vi "M1M3SupportSimulator.vi"   [LabVIEW 2016]
uses:
  Common_FPGA_HealthAndStatus/DataTypes/HealthAndStatusSettings.ctl
  Common_FPGA_Timestamp/DataTypes/TimestampSettings.ctl
  Common_FPGA_HealthAndStatus/DataTypes/HealthAndStatusFIFOCopySettings.ctl
  Common_FPGA_Modbus/DataTypes/ModbusPortSettings.ctl
  FPGAMockHPILC/DataTypes/MockHPILCSettings.ctl
  Common_FPGA_Modbus/DataTypes/ModbusCRCSettings.ctl
  FPGAMockFAILC/DataTypes/MockFAILC1Settings.ctl
  FPGAMockFAILC/DataTypes/MockFAILC2Settings.ctl
  FPGAMockFAILC/DataTypes/MockFAILC3Settings.ctl
  FPGAMockFAILC/DataTypes/MockFAILC4Settings.ctl
  FPGAMockInclin/DataTypes/MockInclinSettings.ctl
  FPGAMockDisplace/DataTypes/MockDisplaceSettings.ctl
  <vilib>/rvi/Emulation/niFpgaGetClockAttributes.vi
  <vilib>/rvi/Emulation/niFpgaSctlEmulationGetInTimedLoop.vi
  <vilib>/rvi/Emulation/niFpgaEmulationReportErrorSimple.vi
  <vilib>/rvi/eio/common/nirviEmuTemplateMethod_errors.vi
  <vilib>/rvi/Emulation/niFpgaCriticalErrorInLSC.vi
  <vilib>/rvi/Emulation/niFpgaEmulationIsFPGAContextNoSignature.vi
  <vilib>/rvi/errors/niFpgaSetErrorForExecOnDevCompSimple.vi
  <vilib>/rvi/eio/common/nirviEmuReportErrorAndStop.vi
  <vilib>/rvi/DataTransferAndStorage/Container/Common/niFpgaContainerGetUniqueNameForEmu.vi
  <vilib>/rvi/FIFO/Fifo_Resource/nirvififoEmulationSetSize.vi
  <vilib>/rvi/FIFO/Fifo_Resource/nirviFifoEmulationQueueMgr.vi
  <instcachedir>/0/nirviFifoEmulationQueueMgr_E5CAEC123FF24DC58D834DCA3CDAA9B5.lvgen/nirviFifoEmulationQueueMgr_E5CAEC123FF24DC58D834DCA3CDAA9B5_007.vi
  <vilib>/Utility/error.llb/Clear Errors.vi
  <vilib>/rvi/FIFO/Fifo_Resource/nirvififoEmulationCreateLock.vi
  <vilib>/rvi/Emulation/niFpgaProcessEmulError.vi
  <vilib>/rvi/FIFO/Fifo_Resource/nirvififoEmulationObtainLock.vi
  <vilib>/rvi/FIFO/Fifo_Resource/nirvififoEmulationReleaseLock.vi
  <vilib>/rvi/occurrence/nirviWaitOnOccurrenceBase.vi
  <vilib>/rvi/errors/nirviReportUnexpectedCaseInternalError.vi
  <vilib>/rvi/errors/nirviReportUnexpectedCaseInternalError (U32).vi
  <vilib>/eio/EIOMethodNode/EIOMethodNode.xnode
  <vilib>/rvi/DataTransferAndStorage/Container/XNode/niFpgaContainer.xnode
  <vilib>/rvi/FIFO/Fifo_Resource/nirvififoEmulationRead.vi
  Common_FPGA_HealthAndStatus/FPGAHealthAndStatus.lvlib
  Common_FPGA_Timestamp/FPGATimestamp.lvlib
  Common_FPGA_Modbus/FPGAModbus.lvlib
  FPGAMockHPILC/FPGAMockHPILC.lvlib
  FPGAMockFAILC/FPGAMockFAILC.lvlib
  FPGAMockInclin/FPGAMockInclin.lvlib
  FPGAMockDisplace/FPGAMockDisplace.lvlib
types:
  T1 = typedef "FPGAMockDisplace.lvlib/MockDisplaceSettings.ctl" = cluster{"BufferUpdateFIFO":refnum<k21>, "DisplaceMeasurementMemory":refnum<k21>}
  T2 = typedef "FPGAMockInclin.lvlib/MockInclinSettings.ctl" = cluster{"ModbusRxDataFIFO":refnum<k21>, "ModbusTxDataFIFO":refnum<k21>, "BufferUpdateFIFO":refnum<k21>, "InclinAngleMemory":refnum<k21>}
  T3 = typedef "FPGAModbus.lvlib/ModbusCRCSettings.ctl" = cluster{"DataFIFO":refnum<k21>, "CalculateFIFO":refnum<k21>, "OutputFIFO":refnum<k21>}
  T4 = typedef "FPGAHealthAndStatus.lvlib/HealthAndStatusFIFOCopySettings.ctl" = cluster{"InternalHealthAndStatusFIFO":refnum<k21>, "SourceHealthAndStatusFIFO":refnum<k21>}
  T5 = typedef "FPGAModbus.lvlib/ModbusPortSettings.ctl" = cluster{"TxPort":refnum<k21>, "TxDataFIFO":refnum<k21>, "TxInternalDataFIFO":refnum<k21>, "TxHealthAndStatusFIFO":refnum<k21>, "RxPort":refnum<k21>, "RxDataFIFO":refnum<k21>, "RxHealthAndStatusFIFO":refnum<k21>, "WaitForRxFrameRegister":refnum<k21>, "BaseHealthAndStatusAddress":u32, "IRQAddress":u8, "TriggerIRQRegister":refnum<k21>, "SoftwareControlledTrigger":refnum<k21>, "TimestampRegister":refnum<k21>, "TxTimestampFIFO":refnum<k21>}
  T6 = typedef "FPGAMockFAILC.lvlib/MockFAILC4Settings.ctl" = cluster{"ModbusTxDataFIFO":refnum<k21>, "Code17Memory":refnum<k21>, "BufferUpdateFIFO":refnum<k21>, "ModbusRxDataFIFO":refnum<k21>, "Code18Memory":refnum<k21>, "Code65Memory":refnum<k21>, "Code66Memory":refnum<k21>, "Code67Memory":refnum<k21>, "Code72Memory":refnum<k21>, "Code80Memory":refnum<k21>, "Code110Memory":refnum<k21>, "CRCDataFIFO":refnum<k21>, "CRCCalculateFIFO":refnum<k21>, "CRCFIFO":refnum<k21>}
  T7 = typedef "FPGAMockFAILC.lvlib/MockFAILC3Settings.ctl" = cluster{"ModbusTxDataFIFO":refnum<k21>, "Code17Memory":refnum<k21>, "BufferUpdateFIFO":refnum<k21>, "ModbusRxDataFIFO":refnum<k21>, "Code18Memory":refnum<k21>, "Code65Memory":refnum<k21>, "Code66Memory":refnum<k21>, "Code67Memory":refnum<k21>, "Code72Memory":refnum<k21>, "Code80Memory":refnum<k21>, "Code110Memory":refnum<k21>, "CRCDataFIFO":refnum<k21>, "CRCCalculateFIFO":refnum<k21>, "CRCFIFO":refnum<k21>}
  T8 = typedef "FPGAMockFAILC.lvlib/MockFAILC2Settings.ctl" = cluster{"ModbusTxDataFIFO":refnum<k21>, "Code17Memory":refnum<k21>, "BufferUpdateFIFO":refnum<k21>, "ModbusRxDataFIFO":refnum<k21>, "Code18Memory":refnum<k21>, "Code65Memory":refnum<k21>, "Code66Memory":refnum<k21>, "Code67Memory":refnum<k21>, "Code72Memory":refnum<k21>, "Code80Memory":refnum<k21>, "Code110Memory":refnum<k21>, "CRCDataFIFO":refnum<k21>, "CRCCalculateFIFO":refnum<k21>, "CRCFIFO":refnum<k21>}
  T9 = typedef "FPGAMockFAILC.lvlib/MockFAILC1Settings.ctl" = cluster{"ModbusTxDataFIFO":refnum<k21>, "Code17Memory":refnum<k21>, "BufferUpdateFIFO":refnum<k21>, "ModbusRxDataFIFO":refnum<k21>, "Code18Memory":refnum<k21>, "Code65Memory":refnum<k21>, "Code66Memory":refnum<k21>, "Code67Memory":refnum<k21>, "Code72Memory":refnum<k21>, "Code80Memory":refnum<k21>, "Code110Memory":refnum<k21>, "CRCDataFIFO":refnum<k21>, "CRCCalculateFIFO":refnum<k21>, "CRCFIFO":refnum<k21>}
  T10 = typedef "FPGAMockHPILC.lvlib/MockHPILCSettings.ctl" = cluster{"ModbusRxDataFIFO":refnum<k21>, "ModbusTxDataFIFO":refnum<k21>, "BufferUpdateFIFO":refnum<k21>, "Code17Memory":refnum<k21>, "Code18Memory":refnum<k21>, "Code65Memory":refnum<k21>, "Code66Memory":refnum<k21>, "Code67Memory":refnum<k21>, "Code72Memory":refnum<k21>, "Code80Memory":refnum<k21>, "Code110Memory":refnum<k21>, "CRCDataFIFO":refnum<k21>, "CRCCalculateFIFO":refnum<k21>, "CRCFIFO":refnum<k21>}
  T11 = typedef "FPGATimestamp.lvlib/TimestampSettings.ctl" = cluster{"TimeSource":refnum<k21>, "TimeRegister":refnum<k21>, "IterationsPerMicrosecond":i16, "UpdateFIFO":refnum<k21>, "HealthAndStatusFIFO":refnum<k21>, "HealthAndStatusAddress":i16, "IterationsPerHealthAndStatusUpdate":i16}
  T12 = typedef "FPGAHealthAndStatus.lvlib/HealthAndStatusSettings.ctl" = cluster{"InternalHealthAndStatusFIFO":refnum<k21>, "HealthAndStatusQueryFIFO":refnum<k21>, "HealthAndStatusResponseFIFO":refnum<k21>, "HealthAndStatusMemory":refnum<k21>, "MemorySize":i32}
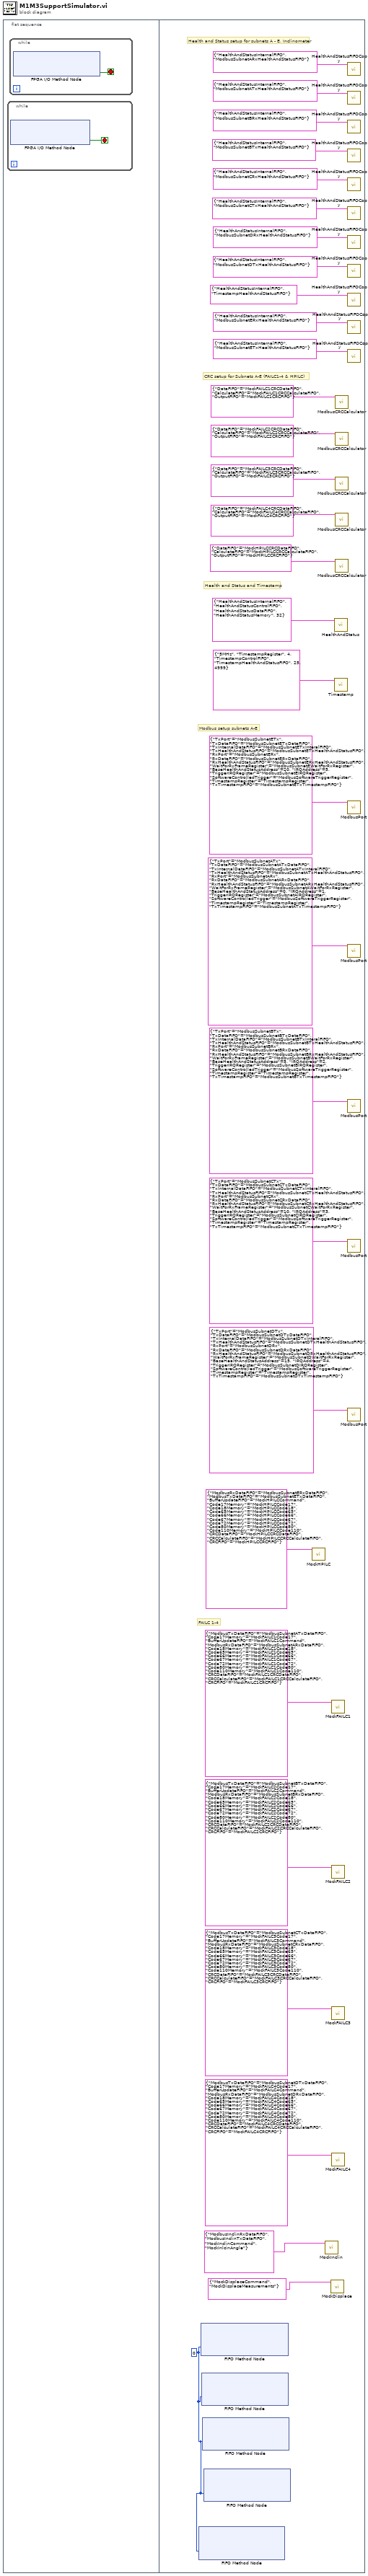
[diagram p0: block diagram]
diagram:
  n1 = flat-sequence {
    frame #0 {
      n2 = while {
        stop <- w2 stop-if-true
        n3 = xnode "FPGA I/O Method Node"() -> ("Ready"=w2:bool)  [unwired: 1 in, 1 out]
      }
      n4 = while {
        stop <- w1 stop-if-true
        n5 = xnode "FPGA I/O Method Node"() -> ("Ready"=w1:bool)  [unwired: 1 in, 1 out]
      }
    }
    frame #1 {
      w5 = 0 ("Timeout")
      # "FAILC 1-4"
      # "Modbus setup subnets A-E"
      # "Health and Status and Timestamp"
      # "CRC setup for Subnets A-E (FAILC1-4 & HPILC)"
      # "Health and Status setup for subnets A - E, Inclinometer"
      n6 = xnode ("FIFO Method Node")("Timeout"=w5) -> ()  [unwired: 1 in, 3 out]
      n7 = xnode ("FIFO Method Node")("Timeout"=w5) -> ()  [unwired: 1 in, 3 out]
      n8 = xnode ("FIFO Method Node")("Timeout"=w5) -> ()  [unwired: 1 in, 3 out]
      n9 = xnode ("FIFO Method Node")("Timeout"=w5) -> ()  [unwired: 1 in, 3 out]
      n10 = xnode ("FIFO Method Node")("Timeout"=w5) -> ()  [unwired: 1 in, 3 out]
      n11 = call "MockHPILC.vi"("MockHPILCSettings"=T10 {"ModbusRxDataFIFO"="ModbusSubnetERxDataFIFO", "ModbusTxDataFIFO"="ModbusSubnetETxDataFIFO", "BufferUpdateFIFO"="MockHPILCCommand", "Code17Memory"="MockHPILCCode17", "Code18Memory"="MockHPILCCode18", "Code65Memory"="MockHPILCCode65", "Code66Memory"="MockHPILCCode66", "Code67Memory"="MockHPILCCode67", "Code72Memory"="MockHPILCCode72", "Code80Memory"="MockHPILCCode80", "Code110Memory"="MockHPILCCode110", "CRCDataFIFO"="MockHPILCCRCDataFIFO", "CRCCalculateFIFO"="MockHPILCCRCCalculateFIFO", "CRCFIFO"="MockHPILCCRCFIFO"}) -> ()  [unwired: 11 in]
      n12 = call "MockInclin.vi"("MockInclinSettings"=T2 {"ModbusRxDataFIFO"="ModbusInclinRxDataFIFO", "ModbusTxDataFIFO"="ModbusInclinTxDataFIFO", "BufferUpdateFIFO"="MockInclinCommand", "InclinAngleMemory"="MockInlcinAngle"}) -> ()  [unwired: 11 in]
      n13 = call "MockDisplace.vi"("MockDisplaceSettings"=T1 {"BufferUpdateFIFO"="MockDisplaceCommand", "DisplaceMeasurementMemory"="MockDisplaceMeasurements"}) -> ()  [unwired: 11 in]
      n14 = call "MockFAILC1.vi"("MockFAILC1Settings"=T9 {"ModbusTxDataFIFO"="ModbusSubnetATxDataFIFO", "Code17Memory"="MockFAILC1Code17", "BufferUpdateFIFO"="MockFAILC1Command", "ModbusRxDataFIFO"="ModbusSubnetARxDataFIFO", "Code18Memory"="MockFAILC1Code18", "Code65Memory"="MockFAILC1Code65", "Code66Memory"="MockFAILC1Code66", "Code67Memory"="MockFAILC1Code67", "Code72Memory"="MockFAILC1Code72", "Code80Memory"="MockFAILC1Code80", "Code110Memory"="MockFAILC1Code110", "CRCDataFIFO"="MockFAILC1CRCDataFIFO", "CRCCalculateFIFO"="MockFAILC1CRCCalculateFIFO", "CRCFIFO"="MockFAILC1CRCFIFO"}) -> ()  [unwired: 11 in]
      n15 = call "MockFAILC2.vi"("MockFAILC2Settings"=T8 {"ModbusTxDataFIFO"="ModbusSubnetBTxDataFIFO", "Code17Memory"="MockFAILC2Code17", "BufferUpdateFIFO"="MockFAILC2Command", "ModbusRxDataFIFO"="ModbusSubnetBRxDataFIFO", "Code18Memory"="MockFAILC2Code18", "Code65Memory"="MockFAILC2Code65", "Code66Memory"="MockFAILC2Code66", "Code67Memory"="MockFAILC2Code67", "Code72Memory"="MockFAILC2Code72", "Code80Memory"="MockFAILC2Code80", "Code110Memory"="MockFAILC2Code110", "CRCDataFIFO"="MockFAILC2CRCDataFIFO", "CRCCalculateFIFO"="MockFAILC2CRCCalculateFIFO", "CRCFIFO"="MockFAILC2CRCFIFO"}) -> ()  [unwired: 11 in]
      n16 = call "MockFAILC3.vi"("MockFAILC3Settings"=T7 {"ModbusTxDataFIFO"="ModbusSubnetCTxDataFIFO", "Code17Memory"="MockFAILC3Code17", "BufferUpdateFIFO"="MockFAILC3Command", "ModbusRxDataFIFO"="ModbusSubnetCRxDataFIFO", "Code18Memory"="MockFAILC3Code18", "Code65Memory"="MockFAILC3Code65", "Code66Memory"="MockFAILC3Code66", "Code67Memory"="MockFAILC3Code67", "Code72Memory"="MockFAILC3Code72", "Code80Memory"="MockFAILC3Code80", "Code110Memory"="MockFAILC3Code110", "CRCDataFIFO"="MockFAILC3CRCDataFIFO", "CRCCalculateFIFO"="MockFAILC3CRCCalculateFIFO", "CRCFIFO"="MockFAILC3CRCFIFO"}) -> ()  [unwired: 11 in]
      n17 = call "MockFAILC4.vi"("MockFAILC4Settings"=T6 {"ModbusTxDataFIFO"="ModbusSubnetDTxDataFIFO", "Code17Memory"="MockFAILC4Code17", "BufferUpdateFIFO"="MockFAILC4Command", "ModbusRxDataFIFO"="ModbusSubnetDRxDataFIFO", "Code18Memory"="MockFAILC4Code18", "Code65Memory"="MockFAILC4Code65", "Code66Memory"="MockFAILC4Code66", "Code67Memory"="MockFAILC4Code67", "Code72Memory"="MockFAILC4Code72", "Code80Memory"="MockFAILC4Code80", "Code110Memory"="MockFAILC4Code110", "CRCDataFIFO"="MockFAILC4CRCDataFIFO", "CRCCalculateFIFO"="MockFAILC4CRCCalculateFIFO", "CRCFIFO"="MockFAILC4CRCFIFO"}) -> ()  [unwired: 11 in]
      n18 = call "HealthAndStatus.vi"("HealthAndStatusSettings"=T12 {"InternalHealthAndStatusFIFO"="HealthAndStatusInternalFIFO", "HealthAndStatusQueryFIFO"="HealthAndStatusControlFIFO", "HealthAndStatusResponseFIFO"="HealthAndStatusDataFIFO", "HealthAndStatusMemory"="HealthAndStatusMemory", "MemorySize"=32}) -> ()  [unwired: 11 in]
      n19 = call "Timestamp.vi"("TimestampSettings"=T11 {"TimeSource"="5MHz", "TimeRegister"="TimestampRegister", "IterationsPerMicrosecond"=4, "UpdateFIFO"="TimestampControlFIFO", "HealthAndStatusFIFO"="TimestampHealthAndStatusFIFO", "HealthAndStatusAddress"=25, "IterationsPerHealthAndStatusUpdate"=4999}) -> ()  [unwired: 11 in]
      n20 = call "ModbusCRCCalculator.vi"("ModbusCRCSettings"=T3 {"DataFIFO"="MockFAILC1CRCDataFIFO", "CalculateFIFO"="MockFAILC1CRCCalculateFIFO", "OutputFIFO"="MockFAILC1CRCFIFO"}) -> ()  [unwired: 11 in]
      n21 = call "ModbusCRCCalculator.vi"("ModbusCRCSettings"=T3 {"DataFIFO"="MockFAILC2CRCDataFIFO", "CalculateFIFO"="MockFAILC2CRCCalculateFIFO", "OutputFIFO"="MockFAILC2CRCFIFO"}) -> ()  [unwired: 11 in]
      n22 = call "ModbusCRCCalculator.vi"("ModbusCRCSettings"=T3 {"DataFIFO"="MockFAILC3CRCDataFIFO", "CalculateFIFO"="MockFAILC3CRCCalculateFIFO", "OutputFIFO"="MockFAILC3CRCFIFO"}) -> ()  [unwired: 11 in]
      n23 = call "ModbusCRCCalculator.vi"("ModbusCRCSettings"=T3 {"DataFIFO"="MockFAILC4CRCDataFIFO", "CalculateFIFO"="MockFAILC4CRCCalculateFIFO", "OutputFIFO"="MockFAILC4CRCFIFO"}) -> ()  [unwired: 11 in]
      n24 = call "ModbusCRCCalculator.vi"("ModbusCRCSettings"=T3 {"DataFIFO"="MockHPILCCRCDataFIFO", "CalculateFIFO"="MockHPILCCRCCalculateFIFO", "OutputFIFO"="MockHPILCCRCFIFO"}) -> ()  [unwired: 11 in]
      n25 = call "HealthAndStatusFIFOCopy.vi"("HealthAndStatusSettingsFIFOCopySettings"=T4 {"InternalHealthAndStatusFIFO"="HealthAndStatusInternalFIFO", "SourceHealthAndStatusFIFO"="ModbusSubnetARxHealthAndStatusFIFO"}) -> ()  [unwired: 11 in]
      n26 = call "HealthAndStatusFIFOCopy.vi"("HealthAndStatusSettingsFIFOCopySettings"=T4 {"InternalHealthAndStatusFIFO"="HealthAndStatusInternalFIFO", "SourceHealthAndStatusFIFO"="ModbusSubnetATxHealthAndStatusFIFO"}) -> ()  [unwired: 11 in]
      n27 = call "HealthAndStatusFIFOCopy.vi"("HealthAndStatusSettingsFIFOCopySettings"=T4 {"InternalHealthAndStatusFIFO"="HealthAndStatusInternalFIFO", "SourceHealthAndStatusFIFO"="ModbusSubnetBRxHealthAndStatusFIFO"}) -> ()  [unwired: 11 in]
      n28 = call "HealthAndStatusFIFOCopy.vi"("HealthAndStatusSettingsFIFOCopySettings"=T4 {"InternalHealthAndStatusFIFO"="HealthAndStatusInternalFIFO", "SourceHealthAndStatusFIFO"="ModbusSubnetBTxHealthAndStatusFIFO"}) -> ()  [unwired: 11 in]
      n29 = call "HealthAndStatusFIFOCopy.vi"("HealthAndStatusSettingsFIFOCopySettings"=T4 {"InternalHealthAndStatusFIFO"="HealthAndStatusInternalFIFO", "SourceHealthAndStatusFIFO"="ModbusSubnetCRxHealthAndStatusFIFO"}) -> ()  [unwired: 11 in]
      n30 = call "HealthAndStatusFIFOCopy.vi"("HealthAndStatusSettingsFIFOCopySettings"=T4 {"InternalHealthAndStatusFIFO"="HealthAndStatusInternalFIFO", "SourceHealthAndStatusFIFO"="ModbusSubnetCTxHealthAndStatusFIFO"}) -> ()  [unwired: 11 in]
      n31 = call "HealthAndStatusFIFOCopy.vi"("HealthAndStatusSettingsFIFOCopySettings"=T4 {"InternalHealthAndStatusFIFO"="HealthAndStatusInternalFIFO", "SourceHealthAndStatusFIFO"="ModbusSubnetDRxHealthAndStatusFIFO"}) -> ()  [unwired: 11 in]
      n32 = call "HealthAndStatusFIFOCopy.vi"("HealthAndStatusSettingsFIFOCopySettings"=T4 {"InternalHealthAndStatusFIFO"="HealthAndStatusInternalFIFO", "SourceHealthAndStatusFIFO"="ModbusSubnetDTxHealthAndStatusFIFO"}) -> ()  [unwired: 11 in]
      n33 = call "HealthAndStatusFIFOCopy.vi"("HealthAndStatusSettingsFIFOCopySettings"=T4 {"InternalHealthAndStatusFIFO"="HealthAndStatusInternalFIFO", "SourceHealthAndStatusFIFO"="TimestampHealthAndStatusFIFO"}) -> ()  [unwired: 11 in]
      n34 = call "ModbusPort.vi"("ModbusPortSettings"=T5 {"TxPort"="ModbusSubnetETx", "TxDataFIFO"="ModbusSubnetETxDataFIFO", "TxInternalDataFIFO"="ModbusSubnetETxInteralFIFO", "TxHealthAndStatusFIFO"="ModbusSubnetETxHealthAndStatusFIFO", "RxPort"="ModbusSubnetERx", "RxDataFIFO"="ModbusSubnetERxDataFIFO", "RxHealthAndStatusFIFO"="ModbusSubnetERxHealthAndStatusFIFO", "WaitForRxFrameRegister"="ModbusSubnetEWaitForRxRegister", "BaseHealthAndStatusAddress"=20, "IRQAddress"=5, "TriggerIRQRegister"="ModbusSubnetEIRQRegister", "SoftwareControlledTrigger"="ModbusSoftwareTriggerRegister", "TimestampRegister"="TimestampRegister", "TxTimestampFIFO"="ModbusSubnetETxTimestampFIFO"}) -> ()  [unwired: 10 in]
      n35 = call "ModbusPort.vi"("ModbusPortSettings"=T5 {"TxPort"="ModbusSubnetATx", "TxDataFIFO"="ModbusSubnetATxDataFIFO", "TxInternalDataFIFO"="ModbusSubnetATxInteralFIFO", "TxHealthAndStatusFIFO"="ModbusSubnetATxHealthAndStatusFIFO", "RxPort"="ModbusSubnetARx", "RxDataFIFO"="ModbusSubnetARxDataFIFO", "RxHealthAndStatusFIFO"="ModbusSubnetARxHealthAndStatusFIFO", "WaitForRxFrameRegister"="ModbusSubnetAWaitForRxRegister", "BaseHealthAndStatusAddress"=0, "IRQAddress"=1, "TriggerIRQRegister"="ModbusSubnetAIRQRegister", "SoftwareControlledTrigger"="ModbusSoftwareTriggerRegister", "TimestampRegister"="TimestampRegister", "TxTimestampFIFO"="ModbusSubnetATxTimestampFIFO"}) -> ()  [unwired: 10 in]
      n36 = call "ModbusPort.vi"("ModbusPortSettings"=T5 {"TxPort"="ModbusSubnetBTx", "TxDataFIFO"="ModbusSubnetBTxDataFIFO", "TxInternalDataFIFO"="ModbusSubnetBTxInteralFIFO", "TxHealthAndStatusFIFO"="ModbusSubnetBTxHealthAndStatusFIFO", "RxPort"="ModbusSubnetBRx", "RxDataFIFO"="ModbusSubnetBRxDataFIFO", "RxHealthAndStatusFIFO"="ModbusSubnetBRxHealthAndStatusFIFO", "WaitForRxFrameRegister"="ModbusSubnetBWaitForRxRegister", "BaseHealthAndStatusAddress"=5, "IRQAddress"=2, "TriggerIRQRegister"="ModbusSubnetBIRQRegister", "SoftwareControlledTrigger"="ModbusSoftwareTriggerRegister", "TimestampRegister"="TimestampRegister", "TxTimestampFIFO"="ModbusSubnetBTxTimestampFIFO"}) -> ()  [unwired: 10 in]
      n37 = call "ModbusPort.vi"("ModbusPortSettings"=T5 {"TxPort"="ModbusSubnetCTx", "TxDataFIFO"="ModbusSubnetCTxDataFIFO", "TxInternalDataFIFO"="ModbusSubnetCTxInteralFIFO", "TxHealthAndStatusFIFO"="ModbusSubnetCTxHealthAndStatusFIFO", "RxPort"="ModbusSubnetCRx", "RxDataFIFO"="ModbusSubnetCRxDataFIFO", "RxHealthAndStatusFIFO"="ModbusSubnetCRxHealthAndStatusFIFO", "WaitForRxFrameRegister"="ModbusSubnetCWaitForRxRegister", "BaseHealthAndStatusAddress"=10, "IRQAddress"=3, "TriggerIRQRegister"="ModbusSubnetCIRQRegister", "SoftwareControlledTrigger"="ModbusSoftwareTriggerRegister", "TimestampRegister"="TimestampRegister", "TxTimestampFIFO"="ModbusSubnetCTxTimestampFIFO"}) -> ()  [unwired: 10 in]
      n38 = call "ModbusPort.vi"("ModbusPortSettings"=T5 {"TxPort"="ModbusSubnetDTx", "TxDataFIFO"="ModbusSubnetDTxDataFIFO", "TxInternalDataFIFO"="ModbusSubnetDTxInteralFIFO", "TxHealthAndStatusFIFO"="ModbusSubnetDTxHealthAndStatusFIFO", "RxPort"="ModbusSubnetDRx", "RxDataFIFO"="ModbusSubnetDRxDataFIFO", "RxHealthAndStatusFIFO"="ModbusSubnetDRxHealthAndStatusFIFO", "WaitForRxFrameRegister"="ModbusSubnetDWaitForRxRegister", "BaseHealthAndStatusAddress"=15, "IRQAddress"=4, "TriggerIRQRegister"="ModbusSubnetDIRQRegister", "SoftwareControlledTrigger"="ModbusSoftwareTriggerRegister", "TimestampRegister"="TimestampRegister", "TxTimestampFIFO"="ModbusSubnetDTxTimestampFIFO"}) -> ()  [unwired: 10 in]
      n39 = call "HealthAndStatusFIFOCopy.vi"("HealthAndStatusSettingsFIFOCopySettings"=T4 {"InternalHealthAndStatusFIFO"="HealthAndStatusInternalFIFO", "SourceHealthAndStatusFIFO"="ModbusSubnetERxHealthAndStatusFIFO"}) -> ()  [unwired: 11 in]
      n40 = call "HealthAndStatusFIFOCopy.vi"("HealthAndStatusSettingsFIFOCopySettings"=T4 {"InternalHealthAndStatusFIFO"="HealthAndStatusInternalFIFO", "SourceHealthAndStatusFIFO"="ModbusSubnetETxHealthAndStatusFIFO"}) -> ()  [unwired: 11 in]
    }
  }
